vi "Background Loop.vi"(8 "error in (no error)":errorcluster, 10 "Action":T1, 11 "Worker in":refnum<class "Worker Actor.lvclass">) -> (0 "error out":errorcluster, 3 "Worker out":refnum<class "Worker Actor.lvclass">, 4 "Result":refnum<class "Acquired Result.lvclass">)   [LabVIEW 2021, in "Worker Actor.lvclass"]
uses:
  Worker Actor.lvclass
  C:/Program Files/National Instruments/LabVIEW 2021/vi.lib/ActorFramework/Actor/Actor.lvclass
  Background Loop Action.ctl
  NHMFL_Core/Libraries/Instruments/Results/Acquired Result/Acquired Result.lvclass
  <vilib>/ActorFramework/Actor/Actor.lvclass/Actor.ctl
  <vilib>/ActorFramework/Message Enqueuer/Message Enqueuer.lvclass/Message Enqueuer.ctl
  Worker Messages/Background Loop Msg/Background Loop Msg.lvclass/Background Loop Msg.ctl
  Worker Messages/Background Loop Msg/Background Loop Msg.lvclass
  C:/Program Files/National Instruments/LabVIEW 2021/vi.lib/ActorFramework/Message/Message.lvclass
  NHMFL_Core/Libraries/Instruments/Instrument Driver/Worker State.ctl
  Worker Actor.lvclass/Worker Actor.ctl
  <vilib>/ActorFramework/Message Enqueuer/Init from Existing Queue.vi
  <vilib>/ActorFramework/Message Enqueuer/Enqueue.vi
  <vilib>/ActorFramework/Message Priority Queue/Priority Enqueue.vi
  <vilib>/ActorFramework/Message Enqueuer/Message Enqueuer.lvclass
  <vilib>/ActorFramework/Actor/Actor.lvclass
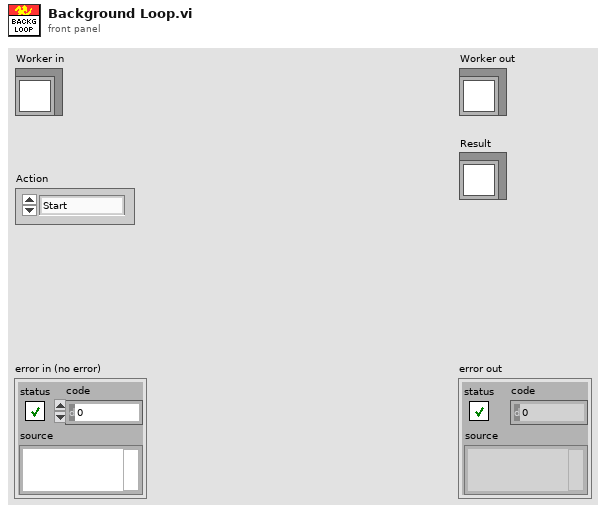
[diagram p1: front panel]
types:
  T1 = typedef "Background Loop Action.ctl" = enum16{"Start", "Continue", "Stop"}
  T2 = typedef "Worker State.ctl" = enum16{"Idle", "Starting", "Working", "Stopping"}
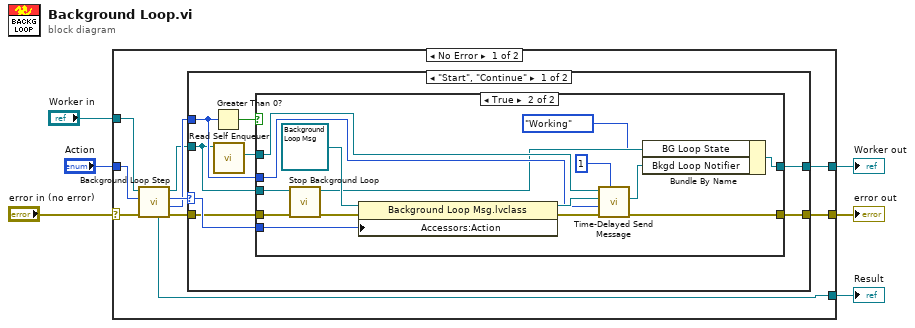
[diagram p0: block diagram]
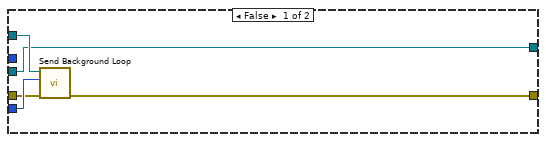
[diagram p2: hidden frame]
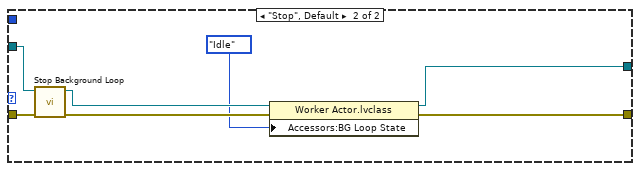
[diagram p3: hidden frame]
diagram:
  n1 = case shown="No Error" "error in (no error)" {
    selector: "error in (no error)" -> [w15 w53]
    tunnel: [w11 w53] -> w5
    tunnel: [w7 w52] -> w3
    tunnel: "Worker in" -> [w16 w52]
    tunnel: "Action" -> [w10 _]
    tunnel: [w9 _] -> w1
    frame No Error {
      n2 = call-dynamic "Background Loop Step.vi"("error in (no error)"=w15, "Action"=w10, "Worker in"=w16) -> ("error out"=w12:errorcluster, "Next step delay"=w13:i32, "Action out"=w14:T1, "Worker out"=w8:refnum<class "Worker Actor.lvclass">, "Result"=w9:refnum<class "Acquired Result.lvclass">)  [unwired: 4 in]
      n3 = case shown="\"Start\", \"Continue\"" w14 {
        selector: w14 -> [w24 _]
        tunnel: w13 -> [w19 _]
        tunnel: w8 -> [w18 w50]
        tunnel: w12 -> [w22 w48]
        tunnel: [w20 w47] -> w11
        tunnel: [w17 w46] -> w7
        frame "Start", "Continue" {
          n4 = Greater Than 0?(x=w19) -> (x > 0?=w23:bool)
          n5 = call <vilib>:"Read Self Enqueuer.vi"("Actor"=w18) -> ("Self Enqueuer"=w21:refnum<class "Message Enqueuer.lvclass">)  [unwired: 10 in]
          n6 = case shown="True" w23 {
            tunnel: w24 -> [w28 w43]
            tunnel: w22 -> [w27 w36]
            tunnel: w21 -> [w29 w38]
            tunnel: [w26 w39] -> w20
            tunnel: w19 -> [_ w41]
            tunnel: w18 -> [w25 w34]
            tunnel: [w25 w32] -> w17
            frame False {
              n7 = call "Send Background Loop.vi"("error in (no error)"=w27, "Action"=w28, "Message Enqueuer"=w29) -> ("error out"=w26:errorcluster)  [unwired: 7 in, 1 out]
            }
            frame True {
              n8 = call-dynamic "Stop Background Loop.vi"("error in (no error)"=w36, "Worker Actor in"=w34) -> ("error out"=w35:errorcluster, "Worker Actor out"=w33:refnum<class "Worker Actor.lvclass">)  [unwired: 8 in]
              n9 = property class="Background Loop Msg.lvclass"(reference=refnum<class "Background Loop Msg.lvclass"> refnum ("Background Loop Msg.lvclass"), error in=w35, "Accessors:Action"=w43) -> (reference out=w42:refnum<class "Background Loop Msg.lvclass">, error out=w40:errorcluster)
              n10 = call <vilib>:"Time-Delayed Send Message.vi"("# Copies (0 = infinite repeat)"=u32 1, "error in (no error)"=w40, "Milliseconds To Wait"=w41, "Message"=w42, "Message Enqueuer"=w38) -> ("error out"=w39:errorcluster, "Delivery Notifier"=w31:refnum<notifier>)  [unwired: 5 in]
              n11 = Bundle By Name(cluster=w33, "BG Loop State"=Worker_State."Working", "Bkgd Loop Notifier"=w31) -> (w32:refnum<class "Worker Actor.lvclass">)
            }
          }
        }
        frame "Stop", Default {
          n12 = call-dynamic "Stop Background Loop.vi"("error in (no error)"=w48, "Worker Actor in"=w50) -> ("error out"=w49:errorcluster, "Worker Actor out"=w51:refnum<class "Worker Actor.lvclass">)  [unwired: 8 in]
          n13 = property class="Worker Actor.lvclass"(reference=w51, error in=w49, "Accessors:BG Loop State"=Worker_State."Idle" ("BG Loop State")) -> (reference out=w46:refnum<class "Worker Actor.lvclass">, error out=w47:errorcluster)
        }
      }
    }
    frame Error {
    }
  }
  "error out" <- w5
  "Worker out" <- w3
  "Result" <- w1
